vi "Actor Core.vi"(8 "error in":errorcluster, 11 "Class Loader in":refnum<class "Class Loader.lvclass">) -> (0 "error out":errorcluster, 3 "Actor out":refnum<class "Actor.lvclass">)   [LabVIEW 2023, in "Class Loader.lvlib" / "Class Loader.lvclass"]
doc: "(<B>Filename</B>: Actor Framework.lvlib:Actor.lvclass:Actor Core.vi)\n\nReceives messages to the actor, reacts to them, and initiates any error handling that may shut the actor down.\n\nDescendant classes may override this VI to append parallel tasks for the actor to complete while it handles messages. Overrides use the Call Parent Class Method node."
uses:
  Class Loader.lvclass
  <vilib>/ActorFramework/Actor/Actor.lvclass
  <vilib>/ActorFramework/Actor/Actor.lvclass/Actor.ctl
  <vilib>/ActorFramework/Message Enqueuer/Message Enqueuer.lvclass/Message Enqueuer.ctl
  Class Loader.lvclass/Class Loader.ctl
  <vilib>/ActorFramework/Message Enqueuer/Init from Existing Queue.vi
  <vilib>/LS Instruments AG/Async Methods Actor/Async Methods Actor/Async Methods Actor/Async Methods Actor.lvclass
  <vilib>/ActorFramework/Message Enqueuer/Message Enqueuer.lvclass
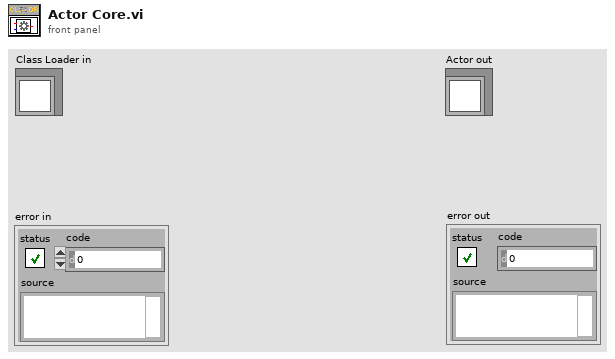
[diagram p1: front panel]
types:
  T1 = typedef "Class Loader.lvlib/Class Loader.lvclass/Load Inputs.ctl" = cluster{"Caller Enqueuer":refnum<class "Message Enqueuer.lvclass">, "Reference Class Path":path, "Class Relative Paths Path":path}
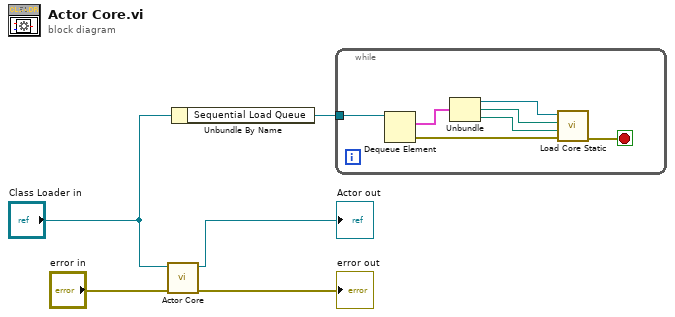
[diagram p0: block diagram]
diagram:
  n1 = call-parent "Actor Core.vi"("error in"="error in", "Actor in"="Class Loader in") -> ("error out"=→"error out":errorcluster, "Actor out"=→"Actor out":refnum<class "Actor.lvclass">)  [unwired: 8 in]
  n2 = Unbundle By Name("Class Loader in") -> ("Sequential Load Queue"=w2:refnum<queue>)
  n3 = while {
    tunnel: w2 -> [w12]
    stop <- w7 stop-if-true
    n4 = Dequeue Element(queue=w12) -> (element=w10:T1, error out=w11:errorcluster)  [unwired: 2 in, 2 out]
    n5 = Unbundle(w10) -> ("Caller Enqueuer"=w6:refnum<class "Message Enqueuer.lvclass">, "Reference Class Path"=w9:path, "Class Relative Paths Path"=w8:path)
    n6 = call "Load Core Static.vi"("error in (no error)"=w11, "Class Relative Paths Path"=w8, "Reference Class Path"=w9, "Message Enqueuer in"=w6) -> ("error out"=w7:errorcluster)  [unwired: 7 in]
  }
